vi "Scheduler.vi"(4 "Settings":cluster{"Numeric":dbl, "Boolean":bool}, 7 "Action":enum16{""}(ring), 8 "error in (no error)":errorcluster, 9 "Inputs 2":cluster{"Numeric":dbl, "Boolean":bool}, 10 "Inputs":cluster{"Numeric":dbl, "Boolean":bool}, 11 "Path In":path) -> (0 "error out":errorcluster, 1 "Outputs 2":cluster{"Numeric":dbl, "Boolean":bool}, 2 "Outputs":cluster{"Numeric":dbl, "Boolean":bool}, 3 "Path Out":path)   [LabVIEW 2018]
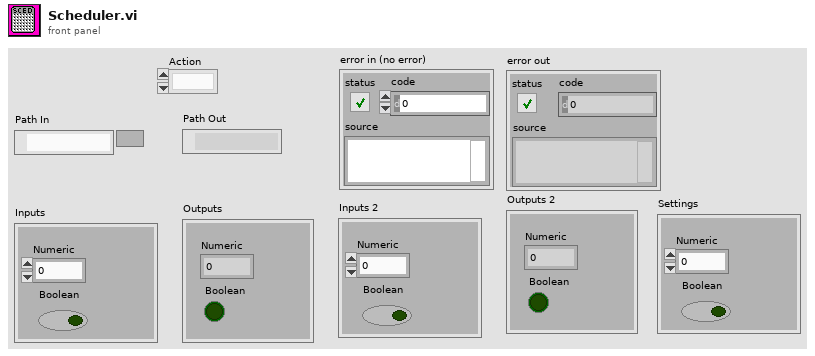
[diagram p1: front panel]
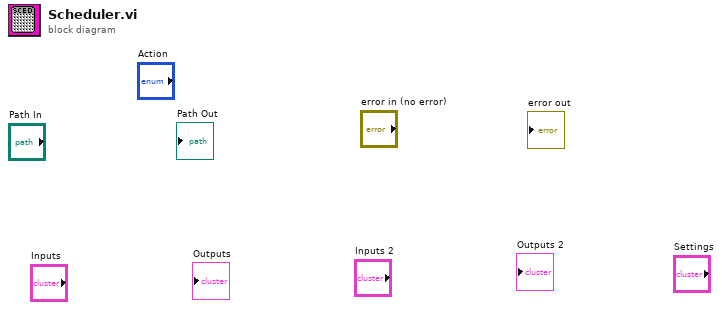
[diagram p0: block diagram]
diagram:
